vi "Status send Error cluster.vi"(0 "error in (no error)":errorcluster, 1 "milliseconds to wait (0)":u32, 5 "Send status msg \"XXX\" or don't wire for no message":string="XXX") -> (6 "error out":errorcluster)   [LabVIEW 2013]
doc: "force to wait data flow through error cluster for set value in ms. \nIf status message wired (not \"XXX\"), sends status message to global variable"
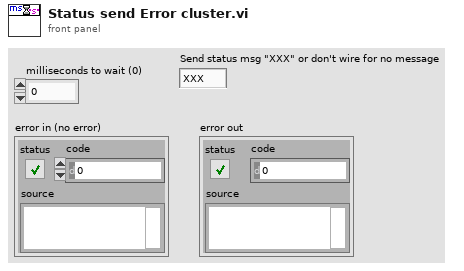
[diagram p1: front panel]
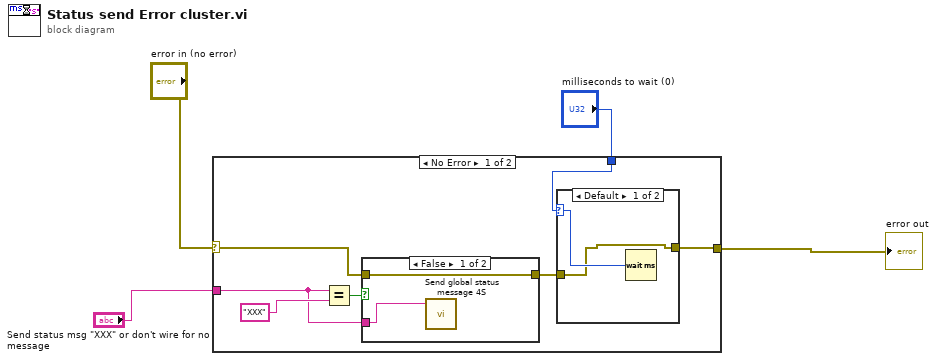
[diagram p0: block diagram]
diagram:
  n1 = case shown="No Error" "error in (no error)" {
    selector: "error in (no error)" -> [w6 w18]
    tunnel: "milliseconds to wait (0)" -> [w8 _]
    tunnel: [w7 w18] -> w4
    tunnel: "Send status msg \"XXX\" or don't wire for no message" -> [w9 _]
    frame No Error {
      n2 = Equal?(x=w9, y="XXX" ("Send status msg \"XXX\" or don't wire for no message")) -> (x = y?=w11:bool)
      n3 = case shown="False" w11 {
        tunnel: w9 -> [w16 _]
        tunnel: w6 -> [w15 w17]
        tunnel: [w15 w17] -> w5
        frame False {
          n4 = call "Send global status message 4S.vi"("TEST Status message"=w16) -> ()  [unwired: 2 in]
        }
        frame True {
        }
      }
      n5 = case shown="Default" w8 {
        selector: w8 -> [w13 _]
        tunnel: [w12 w14] -> w7
        tunnel: w5 -> [w12 w14]
        frame Default {
          n6 = Wait (ms)(milliseconds to wait=w13) -> ()  [unwired: 1 out]
        }
        frame 0 {
        }
      }
    }
    frame Error {
    }
  }
  "error out" <- w4
